vi "Octave Test if Active.vi"(8 "error in (no error)":errorcluster) -> (0 "error out":errorcluster, 2 "responding (if no error)":bool)   [LabVIEW 2020]
doc: "Change octave path, add paths to WAC data processing."
uses:
  Globals for GOLPI.vi
  external libraries/GOLPI 0.7.3.1 source distribution LV 20.0 32 bit/GOLPI library.lvlib
panel:
  out "read buffer":string
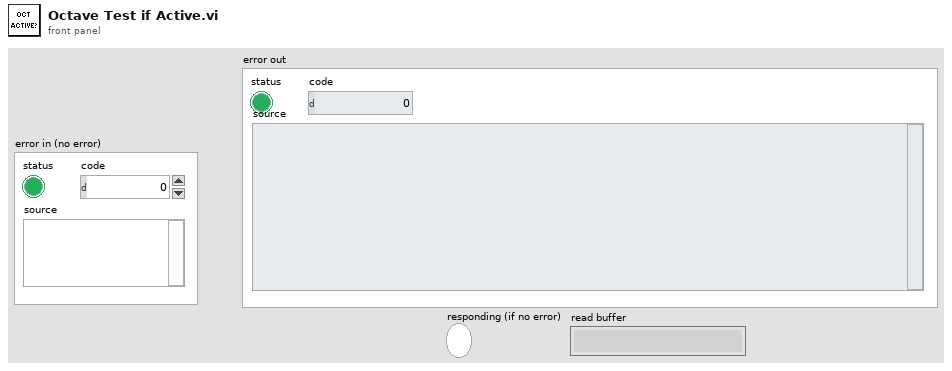
[diagram p1: front panel]
types:
  T1 = typedef "GOLPI library.lvlib/GOLPI reference Type Def.ctl" = cluster{"pipe handle":T2, "fast read timeout [ms]":u32, "fast read settle time [ms]":u32, "fast read to multiple [ms]":u32, "max elements per input line":u32, "slow read timeout [ms]":u32, "stdin double format specifier":string, "max elements per stdout output column":u32, "console mode bitstream":bool, "bitstream first read timeout [ms]":u32, "bitstream read timeout [ms]":u32, "struct transfer possible":bool, "matlab mode":bool}
  T2 = typedef "LV Process library.lvlib/Pipe Handle.ctl" = cluster{"lv_proc.dll file path":path, "process instance handle":u32[], "debug mode":bool, "debug data":cluster{"time":timestamp, "stdin":bool, "data":string}[]}
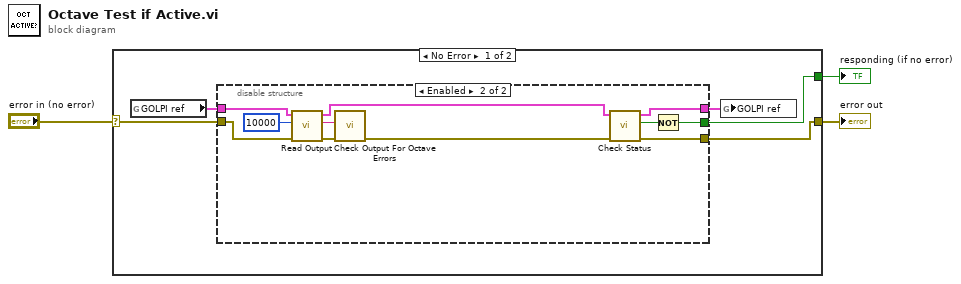
[diagram p0: block diagram]
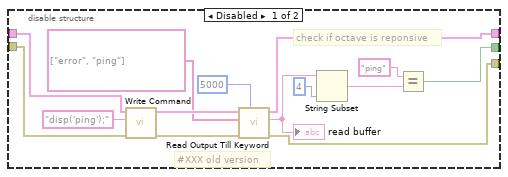
[diagram p2: hidden frame]
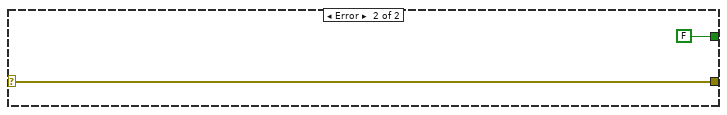
[diagram p3: hidden frame]
diagram:
  n1 = case shown="No Error" "error in (no error)" {
    selector: "error in (no error)" -> [w8 w35]
    tunnel: [w7 w35] -> w3
    tunnel: [w6 FALSE ("status")] -> w1
    frame No Error {
      n2 = global read "Globals for GOLPI.vi" "GOLPI ref"() -> (w4:T1)
      n3 = disable-structure shown="Enabled" {
        disable-tunnel: w8 -> [w17 w28]
        disable-tunnel: [w16 w33] -> w7
        disable-tunnel: [w11 w30] -> w6
        disable-tunnel: [w10 w32] -> w5
        disable-tunnel: w4 -> [w9 w26]
        frame Disabled {
          # "#XXX old version"
          # "check if octave is reponsive"
          n4 = call "Write Command.vi"("error in"=w17, "command"="disp('ping');" ("format string"), "GOLPI ref. in"=w9) -> ("error out"=w22:errorcluster, "GOLPI ref. out"=w21:T1)  [unwired: 7 in]
          n5 = call "Read Output Till Keyword.vi"("timeout [ms]"=u32 5000, "error in"=w22, "keywords"=string[] ["error", "ping"], "GOLPI ref. in"=w21) -> ("error out"=w16:errorcluster, "read buffer"=w15:string, "GOLPI ref. out"=w10:T1)  [unwired: 4 in, 1 out]
          "read buffer" <- w15
          n6 = String Subset(string=w15, length (rest)=4 ("length (rest)")) -> (substring=w13:string)  [unwired: 1 in]
          n7 = Equal?(x="ping", y=w13) -> (x = y?=w11:bool)
        }
        frame Enabled {
          n8 = call "Read Output.vi"("error in"=w28, "byte count"=10000, "GOLPI ref. in"=w26) -> ("error out"=w27:errorcluster, "read buffer"=w24:string, "GOLPI ref. out"=w25:T1)  [unwired: 5 in, 1 out]
          n9 = call "Check Output For Octave Errors.vi"("error in"=w27, "read buffer"=w24) -> ("error out"=w29:errorcluster)  [unwired: 9 in]
          n10 = call "Check Status.vi"("error in"=w29, "GOLPI ref. in"=w25) -> ("error out"=w33:errorcluster, "exited?"=w31:bool, "GOLPI ref. out"=w32:T1)  [unwired: 7 in]
          n11 = Not(x=w31) -> (.not. x?=w30:bool)
        }
      }
      n12 = global write "Globals for GOLPI.vi" "GOLPI ref"(w5) -> ()
    }
    frame Error {
    }
  }
  "error out" <- w3
  "responding (if no error)" <- w1
